vi "Core Write DAQ DVR FIFO.vi"(6 "FIFO Timestamps":T1, 8 "error in (no error)":errorcluster, 9 "Timeout (ms)":i32=100, 10 "Data In":refnum<data-value>[](array[refnum]), 11 "CIFTag in":refnum<class "CIF_NIChn_Fifo_DAQ.lvclass">) -> (0 "error out":errorcluster, 1 "timed out?":bool, 2 "Data Out":refnum<data-value>[](array[refnum]), 3 "CIFTag out":refnum<class "CIF_NIChn_Fifo_DAQ.lvclass">)   [LabVIEW 2021, in "CIF_NIChn_Fifo_DAQ.lvclass"]
uses:
  CIF_NIChn_Fifo_DAQ.lvclass
  D:/dev/Packages/Channel_Manager/src/CIFChannels/CIFChannels.lvclass
  D:/dev/Packages/Channel_Manager/src/CIF_NIChn/NIChn/CIF_NIChn.lvclass
  ChannelCommon/typedef/TimeStamps.ctl
  ChannelCommon/typedef/Datatype Waveform.ctl
  CIF_NIChn_Fifo_DAQ.lvclass/CIF_NIChn_Fifo_DAQ.ctl
  CIFChannels/CIFChannels.lvclass/CIFChannels.ctl
  NIChn/CIF_NIChn.lvclass/CIF_NIChn.ctl
  CIFChannels/Accessors/Read FIFO Header.vi
  ChannelCommon/CIFFIFO/Flatten/DVR Flatten.vi
  <vilib>/CIFChannels/SubVIs/Get dll Path.vi
  <vilib>/CIF Foundation/CIF Utilities/DataTypes/Flatten U64.vi
  CIFChannels/Utilities/Create Flattened FIFO Header.vi
  ChannelCommon/Utilities/Flatten Header.vi
  CIFChannels/Utilities/Update FIFO Header.vi
  <vilib>/CIF Foundation/CIF Utilities/DataTypes/Flatten I64.vi
  <vilib>/CIF Foundation/CIF Utilities/Time/System Time/Get System Time.vi
  <vilib>/CIF Foundation/CIF Utilities/Time/System Time/LabVIEW Time to TAI Time.vi
  NIChn/CIF_NIChn.lvclass
  <vilib>/CIFChannels/CIFChannelCore.lvlib
  ChannelCommon/ChannelCommon.lvlib
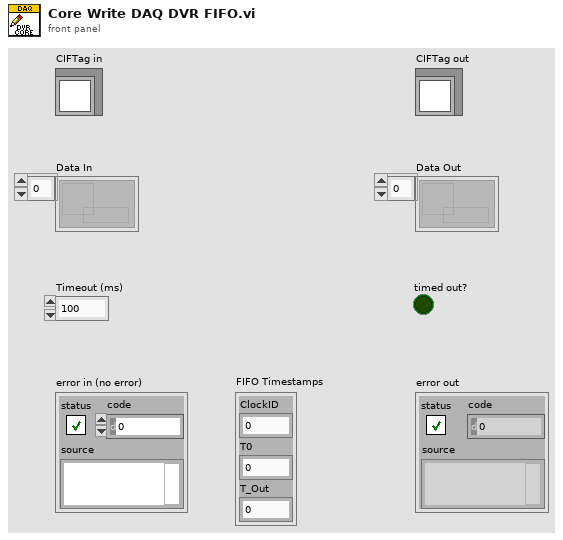
[diagram p1: front panel]
types:
  T1 = typedef "ChannelCommon.lvlib/TimeStamps.ctl" = cluster{"ClockID":u8, "T0":i64, "T_Out":i64}
  T2 = typedef "ChannelCommon.lvlib/FIFO Header.ctl" = cluster{"Length":u64, "T0":i64, "T_Out":i64, "T_Tx":i64, "Ctr":u64, "ClockID":u8}
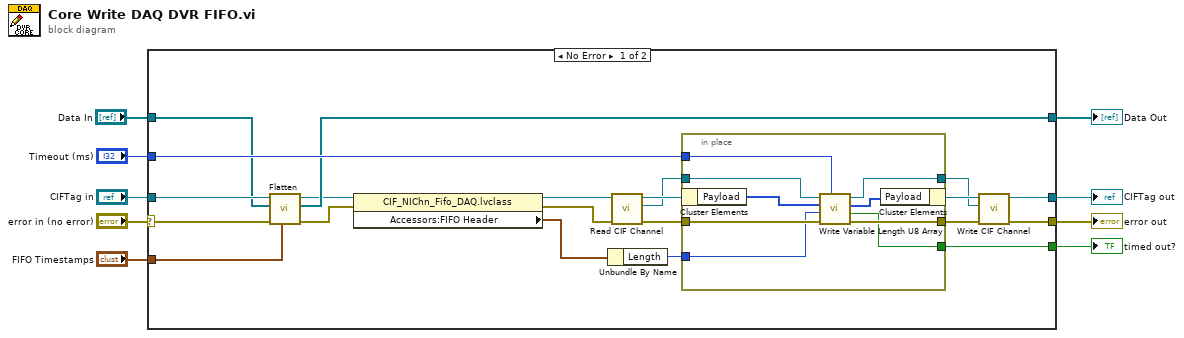
[diagram p0: block diagram]
diagram:
  n1 = case shown="No Error" "error in (no error)" {
    selector: "error in (no error)" -> [w25 w42]
    tunnel: [w27 w42] -> w8
    tunnel: [w29 w41] -> w6
    tunnel: "CIFTag in" -> [w26 w41]
    tunnel: [w30 _] -> w5
    tunnel: "Timeout (ms)" -> [w28 _]
    tunnel: [w24 w40] -> w1
    tunnel: "Data In" -> [w23 w40]
    tunnel: "FIFO Timestamps" -> [w22 _]
    frame No Error {
      n2 = call "Flatten.vi"("FIFO Timestamps"=w22, "error in (no error)"=w25, "Data In"=w23, "CIFTag in"=w26) -> ("error out"=w15:errorcluster, "Data Out"=w24:refnum<data-value>[], "CIFTag out"=w14:refnum<class "CIF_NIChn_Fifo_DAQ.lvclass">)  [unwired: 5 in]
      n3 = property class="CIF_NIChn_Fifo_DAQ.lvclass"(reference=w14, error in=w15) -> (reference out=w13:refnum<class "CIF_NIChn_Fifo_DAQ.lvclass">, error out=w10:errorcluster, "Accessors:FIFO Header"=w12:T2)
      n4 = Unbundle By Name(w12) -> ("Length"=w11:u64)
      n5 = call "Read CIF Channel.vi"("error in (no error)"=w10, "CIFTag in"=w13) -> ("error out"=w20:errorcluster, "CIF Channel"=w17:refnum<k21>, "CIFTag out"=w21:refnum<class "CIF_NIChn_Fifo_DAQ.lvclass">)  [unwired: 7 in]
      n6 = in-place {
        in-place-border: w20 -> [w39]
        in-place-border: [w38] -> w18
        in-place-border: [w37] -> w30
        in-place-border: w17 -> [w36]
        in-place-border: [w35] -> w16
        in-place-border: w28 -> [w34]
        in-place-border: w11 -> [w32]
        n7 = in-place-cluster #1(w21) -> ("Payload"=w33:u8[])
        n8 = call <vilib>:"Write Variable Length U8 Array.vi"("Timeout (ms)"=w34, "error in"=w39, "numElements"=w32, "U8 Array in"=w33, "CIF Channel in"=w36) -> ("error out"=w38:errorcluster, "Timed out?"=w37:bool, "U8 Array out"=w31:u8[], "CIF Channel out"=w35:refnum<k21>)  [unwired: 3 in]
        n9 = in-place-cluster #1("Payload"=w31) -> (w19:refnum<class "CIF_NIChn_Fifo_DAQ.lvclass">)
      }
      n10 = call "Write CIF Channel.vi"("error in (no error)"=w18, "CIF Channel"=w16, "CIFTag in"=w19) -> ("error out"=w27:errorcluster, "CIFTag out"=w29:refnum<class "CIF_NIChn_Fifo_DAQ.lvclass">)  [unwired: 7 in]
    }
    frame Error {
    }
  }
  "error out" <- w8
  "CIFTag out" <- w6
  "timed out?" <- w5
  "Data Out" <- w1
